vi "Set_and_Get.vi"(0 "error in (no error)":errorcluster) -> (2 "error out":errorcluster, 3 "Amplitude":dbl, 4 "Phase Shift":dbl)   [LabVIEW 2010]
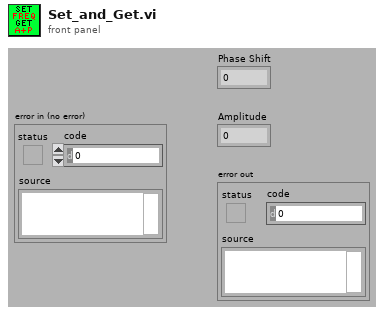
[diagram p1: front panel]
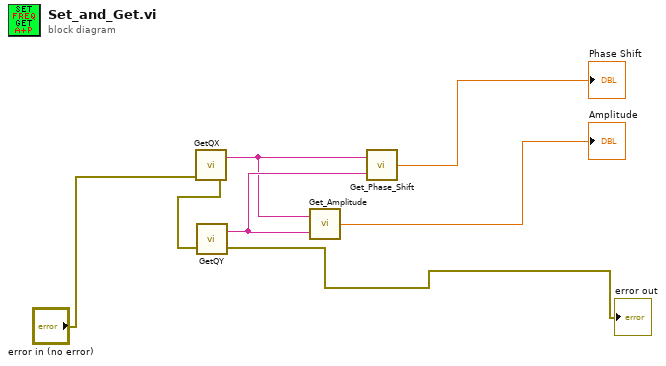
[diagram p0: block diagram]
diagram:
  n1 = call "GetQX.vi"("error in"="error in (no error)") -> ("error out"=w5:errorcluster, "data"=w1:string)  [unwired: 1 in]
  n2 = call "GetQY.vi"("error in"=w5) -> ("error out"=→"error out":errorcluster, "data"=w2:string)  [unwired: 1 in]
  n3 = call "Get_Amplitude.vi"("Data QY"=w2, "Data QX"=w1) -> ("Numeric"=→"Amplitude":dbl)
  n4 = call "Get_Phase_Shift.vi"("Data QY"=w2, "Data QX"=w1) -> ("Numeric"=→"Phase Shift":dbl)
